vi "Set From Result Row.vi"(8 "error in (no error)":errorcluster, 10 "Result Row":refnum<class "Result Row.lvclass">, 11 "Entity in":refnum<class "Entity.lvclass">) -> (0 "error out":errorcluster, 3 "Entity out":refnum<class "Entity.lvclass">)   [LabVIEW 2020, in "Conditu2.lvlib" / "Entity.lvclass"]
uses:
  Entity.lvclass
  Result Row/Result Row.lvclass
  Columns/ID/ID.lvclass
  Result Row/Result Row.lvclass/Result Row.ctl
  Columns/ID/ID.lvclass/ID.ctl
  Entity.lvclass/Entity.ctl
  Update ID.vi
  Columns/ID/Set.vi
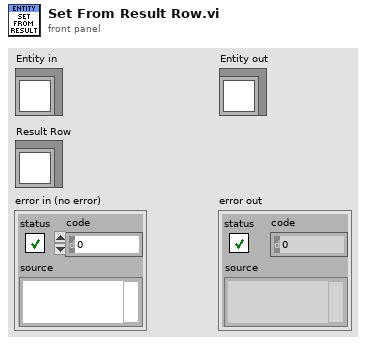
[diagram p1: front panel]
types:
  T1 = typedef "Conditu2.lvlib/Entity ID.ctl" = i64
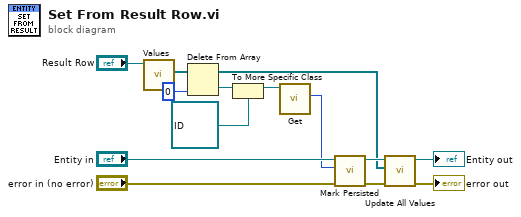
[diagram p0: block diagram]
diagram:
  n1 = call "Values.vi"("Result Row in"="Result Row") -> ("Value"=w12:refnum<class "Type.lvclass">[])  [unwired: 10 in]
  n2 = Delete From Array(array=w12, index=0) -> (deleted portion=w9:refnum<class "Type.lvclass">, array with subset deleted=w3:refnum<class "Type.lvclass">[])  [unwired: 1 in]
  n3 = To More Specific Class(target class=refnum<class "ID.lvclass"> refnum ("Conditum:Columns:ID.lvclass"), reference=w9) -> (specific class reference=w7:refnum<class "ID.lvclass">)  [unwired: 1 in, 1 out]
  n4 = call "Get.vi"("ID in"=w7) -> ("Entity ID"=w6:T1)  [unwired: 10 in]
  n5 = call "Mark Persisted.vi"("Entity ID"=w6, "Entity in"="Entity in") -> ("Entity out"=w4:refnum<class "Entity.lvclass">)  [unwired: 9 in]
  n6 = call-dynamic "Update All Values.vi"("error in (no error)"="error in (no error)", "Values"=w3, "Entity in"=w4) -> ("error out"=→"error out":errorcluster, "Entity out"=→"Entity out":refnum<class "Entity.lvclass">)  [unwired: 7 in]
